vi "Type.vi"(8 "error in (no error)":errorcluster, 11 "Packet in":refnum<class "Packet.lvclass">) -> (0 "error out":errorcluster, 2 "Type":T1, 3 "Packet out":refnum<class "Packet.lvclass">)   [LabVIEW 2020, in "Packet.lvclass"]
uses:
  Packet.lvclass
  Packet.lvclass/Packet.ctl
  Type.ctl
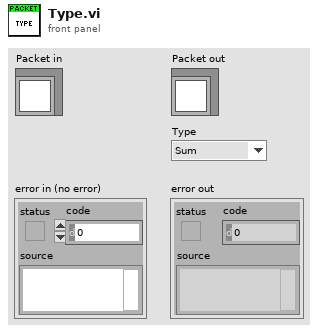
[diagram p1: front panel]
types:
  T1 = typedef "Type.ctl" = enum8{"Sum", "Product", "Minimum", "Maximum", "Literal", "Greater", "Less", "Equal"}
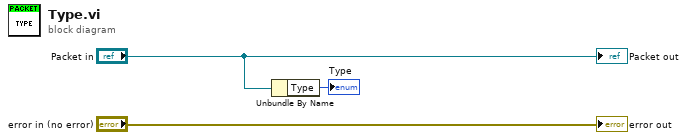
[diagram p0: block diagram]
diagram:
  n1 = Unbundle By Name("Packet in") -> ("Type"=→"Type":T1)
  "error out" <- "error in (no error)"
  "Packet out" <- "Packet in"
